vi "HMI.vi"(8 "error in (no error)":errorcluster caption="entrée d'erreur (pas d'erreur)", 11 "Popup Operator_Input Batch In":refnum<class "Class Popup Operator_Input QR_P2056.lvclass">) -> (0 "error out":errorcluster caption="sortie d'erreur", 1 "Input":string="Attente \nvalidation", 2 "Operator_Selection":bool, 3 "Popup Operator_Input Batch In":refnum<class "Class Popup Operator_Input QR_P2056.lvclass">)   [LabVIEW 2020, in "Library Instrument & Equipement.lvlib" / "Library Popup.lvlib" / "Class Popup Operator_Input QR_P2056.lvclass"]
uses:
  Class Popup Operator_Input QR_P2056.lvclass
  C:/Users/ngarcin/OneDrive - Altyor/Standard TB/Suite TB45/Class/Popup/Class Popup (Main)/Class Popup (Main).lvclass
  Commun VI/TypeDef/Variable Printable.ctl
  JSON API/JSON Value/Set from JSON string.vi
  JSON API/JSON Value/JSON Value.lvclass
  Class Popup (Main)/Class Popup (Main).lvclass
  JSON API/Variant JSON/Variant JSON.lvlib
  JSON API/Get Polymorphic/JSON GetSet.lvlib
  Commun VI/Library Commun.lvlib
panel:
  in  "Bouton NOK":bool
  in  "Input OP":string="Attente \nvalidation"
  in  "Bouton OK":bool
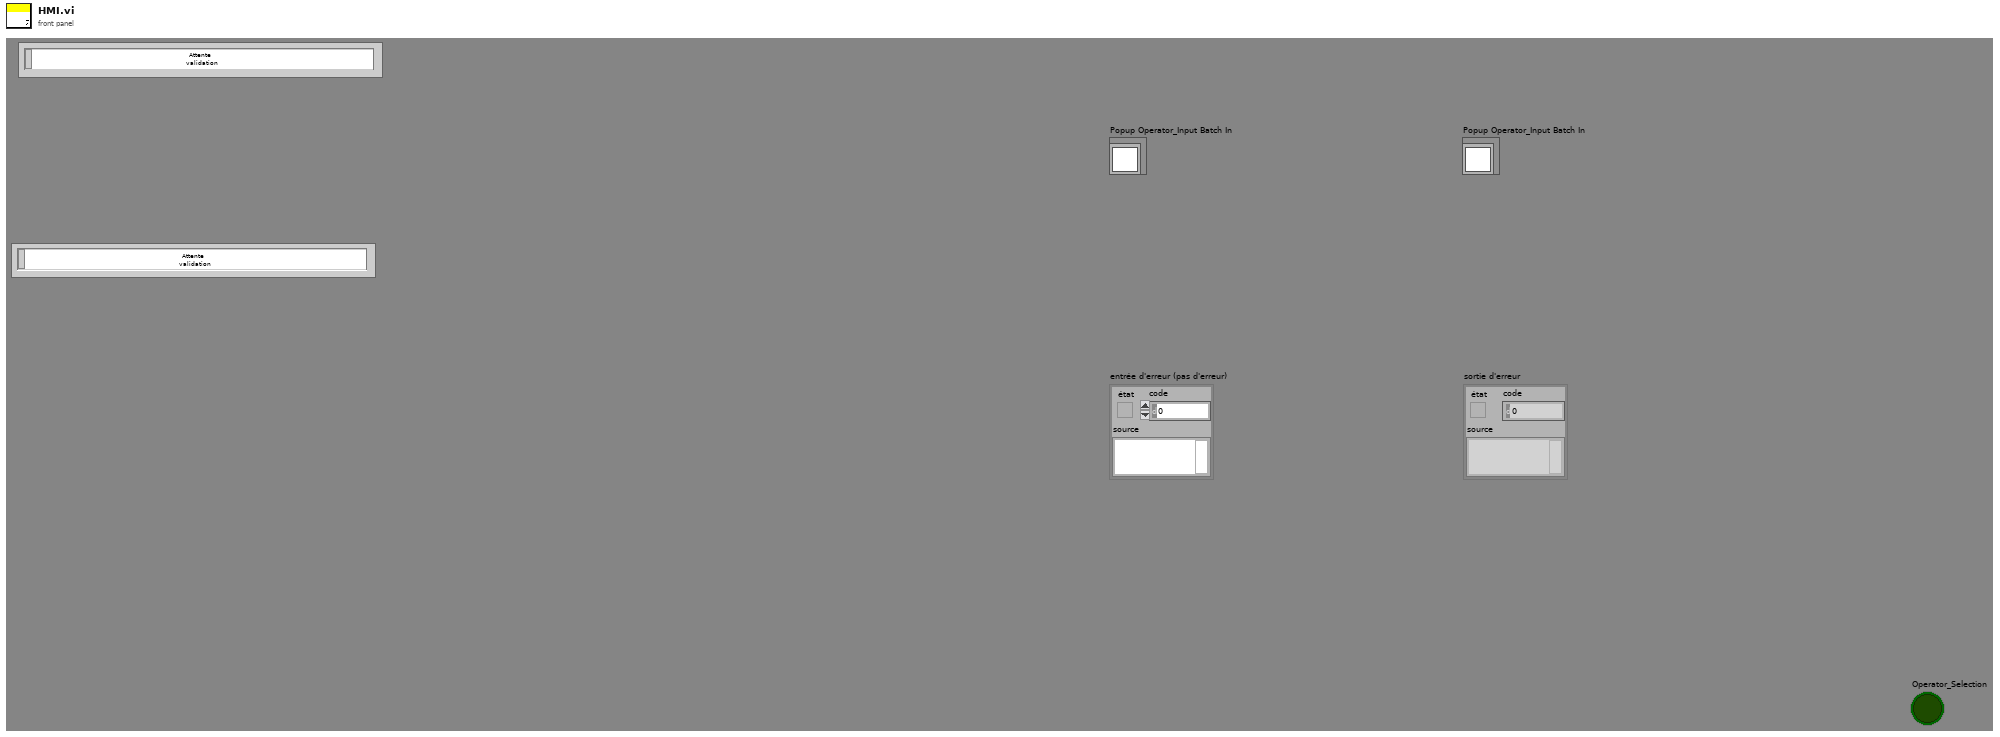
[diagram p1: front panel]
types:
  T1 = enum32{"Invalid", "Standard", "Closed", "Hidden", "Minimized", "Maximized"}
  T2 = typedef "Variable Printable.ctl" = string
  T3 = enum16{"Get Variable", "Get All Variables", "Set Variable", "Delete Variable", "Delete All Variable"}
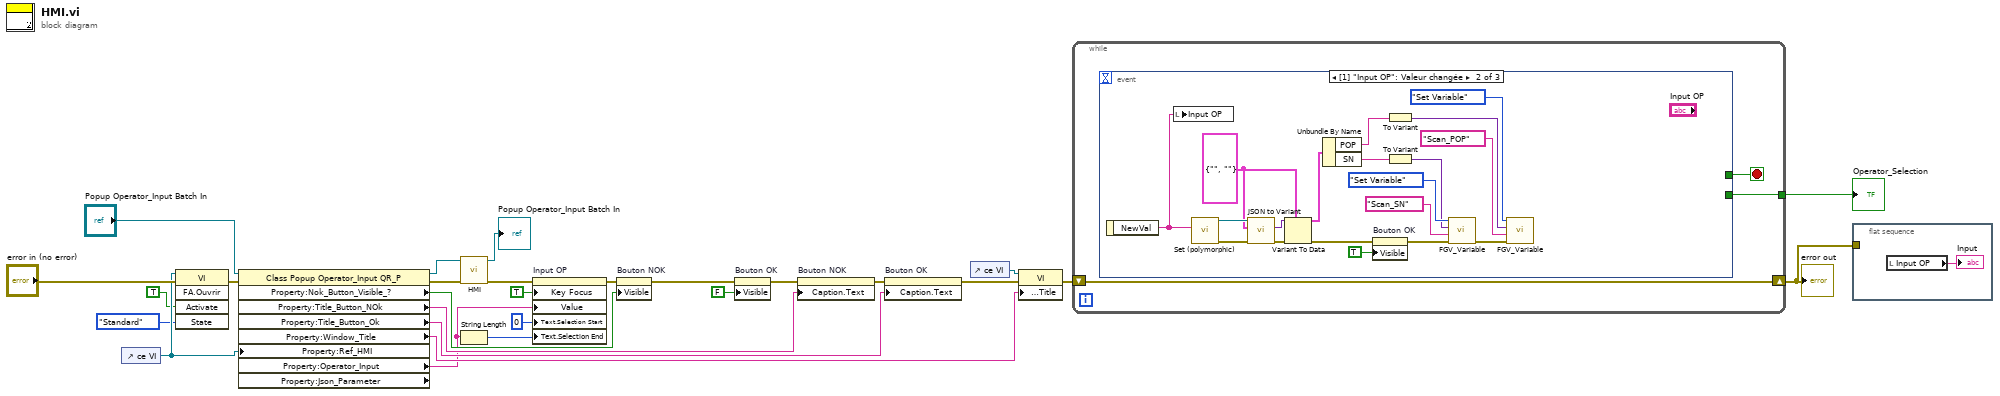
[diagram p0: block diagram]
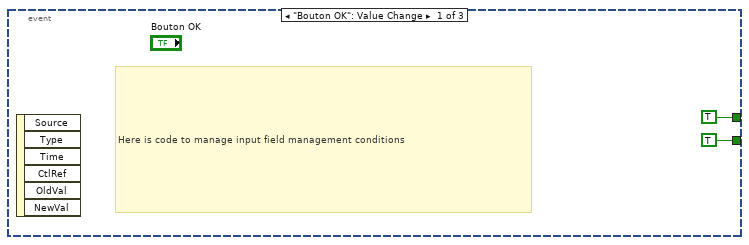
[diagram p2: hidden frame]
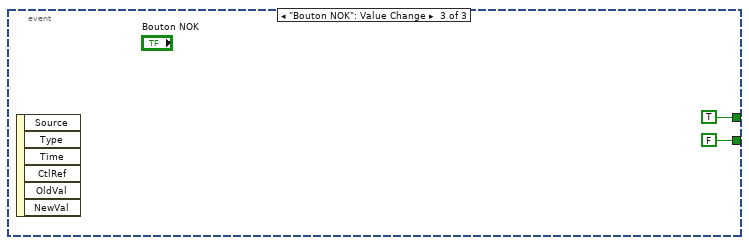
[diagram p3: hidden frame]
diagram:
  n1 = control-ref of="ce VI"() -> (w7:refnum<vi>)
  n2 = invoke class="VI" method="FA.Ouvrir"(reference=w7, error in="error in (no error)", "Activate"=TRUE ("Fenêtre face-avant:Au premier plan"), "State"=T1."Standard" ("État")) -> (error out=w6:errorcluster)  [unwired: 1 in, 4 out]
  n3 = property class="Class Popup Operator_Input QR_P" props=["Property:Nok_Button_Visible_?", "Property:Title_Button_NOk", "Property:Title_Button_Ok", "Property:Window_Title", "Property:Ref_HMI", "Property:Operator_Input", "Property:Json_Parameter"](reference="Popup Operator_Input Batch In", error in=w6, "Property:Ref_HMI"=w7) -> (reference out=w23:refnum<class "Class Popup Operator_Input QR_P2056.lvclass">, error out=w3:errorcluster, "Property:Nok_Button_Visible_?"=w28:bool, "Property:Title_Button_NOk"=w22:string, "Property:Title_Button_Ok"=w20:string, "Property:Window_Title"=w25:string, "Property:Operator_Input"=w12:string)  [unwired: 1 out]
  n4 = call-parent "HMI.vi"("error in (no error)"=w3, "Class Popup (Main) en entrée"=w23) -> ("error out"=w1:errorcluster, "Class Popup (Main) en sortie"=→"Popup Operator_Input Batch In":refnum<class "Class Popup Operator_Input QR_P2056.lvclass">)  [unwired: 6 in, 2 out]
  n5 = String Length(string=w12) -> (length=w14:i32)
  n6 = property on="Input OP" class="Ch"(error in=w1, "Key Focus"=TRUE ("Focus clavier"), "Value"=w12, "Text.Selection Start"=u32 0 ("Texte.Sélection:Début"), "Text.Selection End"=w14) -> (error out=w2:errorcluster)  [unwired: 1 in, 1 out]
  n7 = property on="Bouton NOK" class="Bool"(error in=w2, "Visible"=w28) -> (error out=w18:errorcluster)  [unwired: 1 in, 1 out]
  n8 = property on="Bouton OK" class="Bool"(error in=w18, "Visible"=FALSE ("Activer ?")) -> (error out=w17:errorcluster)  [unwired: 1 in, 1 out]
  n9 = property on="Bouton NOK" class="Bool"(error in=w17, "Caption.Text"=w22) -> (error out=w21:errorcluster)  [unwired: 1 in, 1 out]
  n10 = property on="Bouton OK" class="Bool"(error in=w21, "Caption.Text"=w20) -> (error out=w15:errorcluster)  [unwired: 1 in, 1 out]
  n11 = control-ref of="ce VI"() -> (w26:refnum<vi>)
  n12 = property class="VI"(reference=w26, error in=w15, "Front Panel.Title"=w25) -> (error out=w24:errorcluster)  [unwired: 1 out]
  n13 = while {
    tunnel: [w29] -> w27
    shift-right: [w30] -> w11
    shift-left: w24 -> [w30]
    stop <- w31 stop-if-true
    n14 = event shown="[1] \"Input OP\": Valeur changée" {
      selector: _ -> [_ _ _]
      dyn-events: _ -> [_ _ _]
      timeout: _ -> [_ _ _]
      tunnel: [TRUE ("Valeur (Signalisation)") _ TRUE ("Valeur (Signalisation)")] -> w31
      tunnel: [TRUE ("Operator_Selection") _ FALSE ("Operator_Selection")] -> w29
      event "Bouton OK": Value Change {
        # "Here is code to manage input field management conditions"
        n15 = event-data() -> ()  [unwired: 1 in, 6 out]
      }
      event "Input OP": Value Change {
        w48 = cluster{"SN":string, "POP":string} {"SN"="", "POP"=""}
        n16 = event-data() -> ("NewVal"=w47:string)  [unwired: 1 in]
        n17 = local write "Input OP"(w47) -> ()
        n18 = call-poly "Set (polymorphic).vi"("JSON stream"=w47) -> ("error out"=w50:errorcluster, "JSON Value out"=w52:refnum<class "JSON Value.lvclass">)  [unwired: 8 in, 1 out]
        n19 = call "JSON to Variant.vi"("error in (no error)"=w50, "Variant (Data Type)"=w48, "JSON Value"=w52) -> ("error out"=w51:errorcluster, "Variant out"=w49:variant)  [unwired: 7 in]
        n20 = Variant To Data(error in=w51, type=w48, Variant=w49) -> (data=w38:cluster{"SN":string, "POP":string}, error out=w45:errorcluster)
        n21 = Unbundle By Name(w38) -> ("POP"=w36:string, "SN"=w34:string)
        n22 = property on="Bouton OK" class="Bool"(error in=w45, "Visible"=TRUE) -> (error out=w40:errorcluster)  [unwired: 1 in, 1 out]
        n23 = To Variant(anything=w36) -> (Variant=w35:variant)
        n24 = To Variant(anything=w34) -> (Variant=w37:variant)
        n25 = call "FGV_Variable.vi"("error in (no error)"=w40, "Variable"=T2 "Scan_SN", "Data In"=w37, "Function"=T3."Set Variable") -> ("error out"=w39:errorcluster)  [unwired: 5 in, 2 out]
        n26 = call "FGV_Variable.vi"("error in (no error)"=w39, "Variable"=T2 "Scan_POP", "Data In"=w35, "Function"=T3."Set Variable") -> ()  [unwired: 5 in, 3 out]
      }
      event "Bouton NOK": Value Change {
        n27 = event-data() -> ()  [unwired: 1 in, 6 out]
      }
    }
  }
  "error out" <- w11
  "Operator_Selection" <- w27
  n28 = flat-sequence {
    tunnel: w11 -> [_]
    frame #0 {
      n29 = local read "Input OP"() -> (→"Input":string)
    }
  }
